vi "Empty.vi"(8 "error in (no error)":errorcluster, 11 "Data ref. in":refnum<data-value>) -> (0 "error out":errorcluster, 3 "Data ref.":refnum<data-value>)   [LabVIEW 2013, in "CameraVision.lvlib" / "CV-Main.lvclass"]
uses:
  CV-Main.lvclass
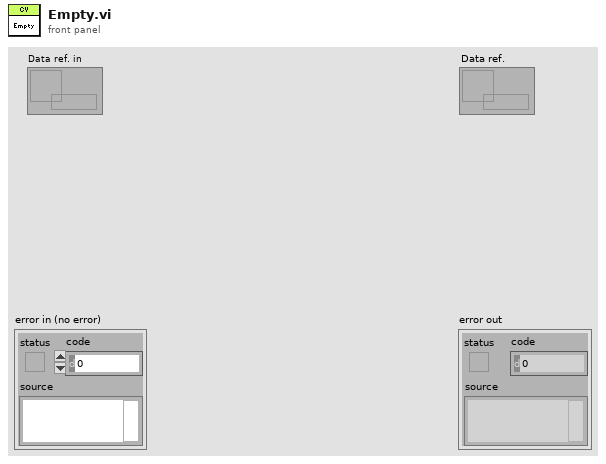
[diagram p1: front panel]
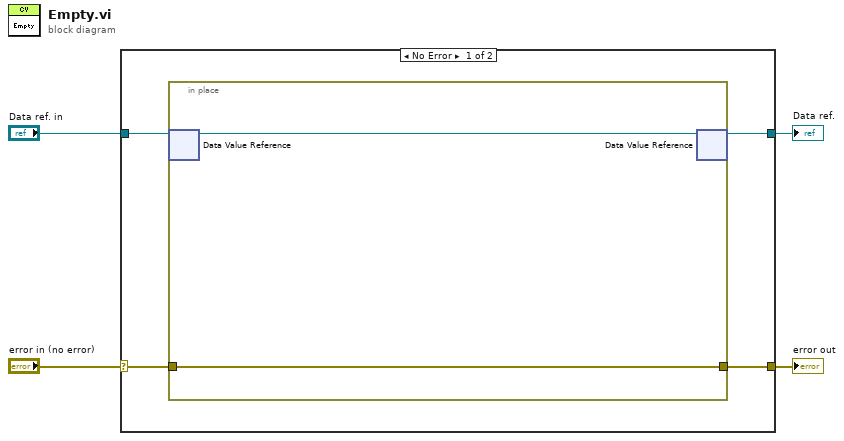
[diagram p0: block diagram]
diagram:
  n1 = case shown="No Error" "error in (no error)" {
    selector: "error in (no error)" -> [w6 w12]
    tunnel: [w5 w12] -> w3
    tunnel: "Data ref. in" -> [w8 w11]
    tunnel: [w7 w11] -> w1
    frame No Error {
      n2 = in-place {
        in-place-border: [w9] -> w5
        in-place-border: w6 -> [w9]
        n3 = in-place-dvr #1(w8) -> (w10:refnum<class "CV-Main.lvclass">)  [unwired: 1 out]
        n4 = in-place-dvr #1(w10) -> (w7:refnum<data-value>)  [unwired: 1 out]
      }
    }
    frame Error {
    }
  }
  "error out" <- w3
  "Data ref." <- w1
